vi "Harris Corner Detection.vi"() -> ()   [LabVIEW 2018]
doc: "Harris Corner Detection: This example is a Harris corner detection example, which can determine which pixels are corners based on the value of the corner response function by setting a threshold. If the corner response function value of a pixel is greater than the threshold and is a local maximum in its surrounding neighborhood, it is considered a corner."
uses:
  vi.lib/VIRobotics/opencv_yiku/ctls/ColorConversionCodes.ctl
  vi.lib/VIRobotics/opencv_yiku/Mat/Create_Mat_8U.vi
  vi.lib/VIRobotics/opencv_yiku/Mat/Mat_8U/set2ddata.vi
  vi.lib/VIRobotics/opencv_yiku/Mat/Mat_8U/Mat_8U.lvclass
  vi.lib/VIRobotics/opencv_yiku/opencv_yiku.lvlib
panel:
  out "max value":sgl
  out "corner":picture
  out "dst":sgl[][](array[numeric])
  out "picture":picture
  # "Overview: Demonstrates how to finish Harris Corner Detection\nRequirements: Windows.\nInstructions: \n1.Run the VI"
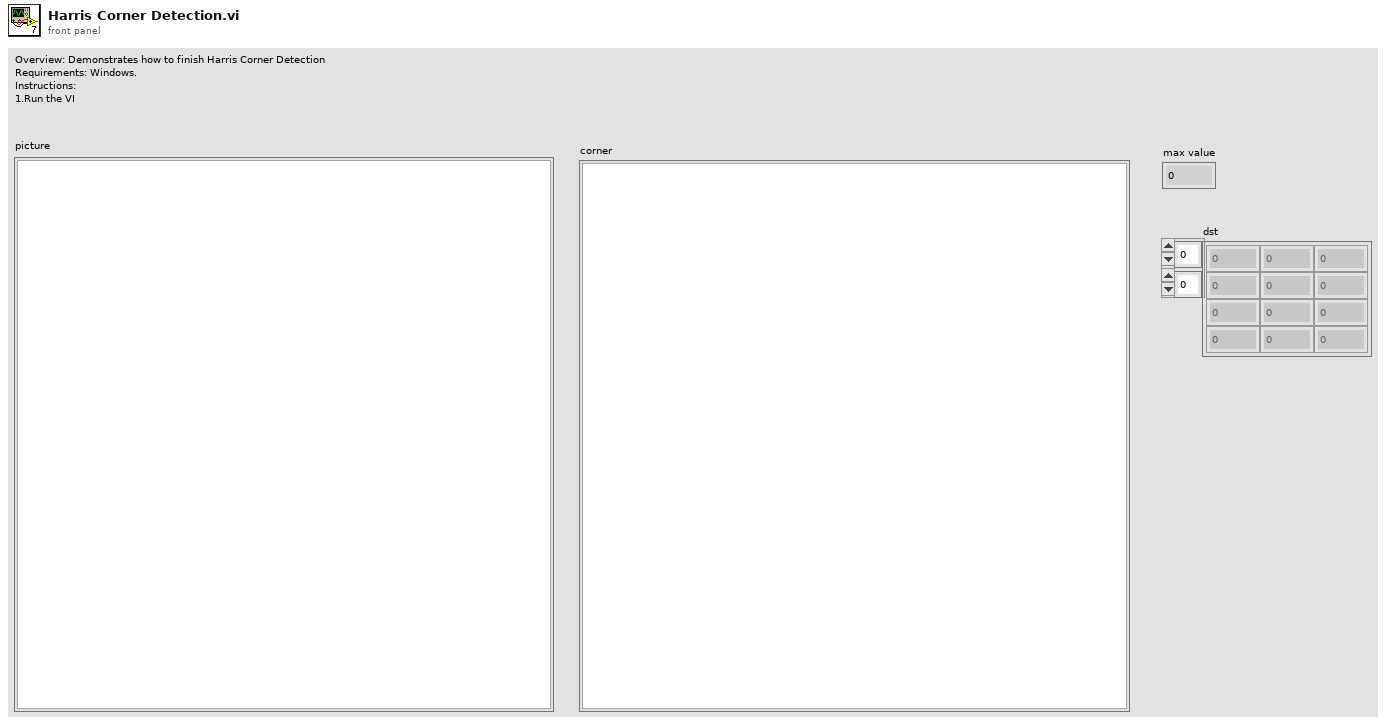
[diagram p1: front panel]
types:
  T1 = typedef "opencv_yiku.lvlib/ColorConversionCodes.ctl" = enum32{"COLOR_BGR2BGRA", "COLOR_BGRA2BGR", "COLOR_BGR2RGBA", "COLOR_RGBA2BGR", "COLOR_BGR2RGB", "COLOR_BGRA2RGBA", "COLOR_BGR2GRAY", "COLOR_RGB2GRAY", "COLOR_GRAY2BGR", "COLOR_GRAY2BGRA", "COLOR_BGRA2GRAY", "COLOR_RGBA2GRAY", "COLOR_BGR2BGR565", "COLOR_RGB2BGR565", "COLOR_BGR5652BGR", "COLOR_BGR5652RGB", "COLOR_BGRA2BGR565", "COLOR_RGBA2BGR565", "COLOR_BGR5652BGRA", "COLOR_BGR5652RGBA", "COLOR_GRAY2BGR565", "COLOR_BGR5652GRAY", "COLOR_BGR2BGR555", "COLOR_RGB2BGR555", "COLOR_BGR5552BGR", "COLOR_BGR5552RGB", "COLOR_BGRA2BGR555", "COLOR_RGBA2BGR555", "COLOR_BGR5552BGRA", "COLOR_BGR5552RGBA", "COLOR_GRAY2BGR555", "COLOR_BGR5552GRAY", "COLOR_BGR2XYZ", "COLOR_RGB2XYZ", "COLOR_XYZ2BGR", "COLOR_XYZ2RGB", "COLOR_BGR2YCrCb", "COLOR_RGB2YCrCb", "COLOR_YCrCb2BGR", "COLOR_YCrCb2RGB", "COLOR_BGR2HSV", "COLOR_RGB2HSV", "42", "43", "COLOR_BGR2Lab", "COLOR_RGB2Lab"}
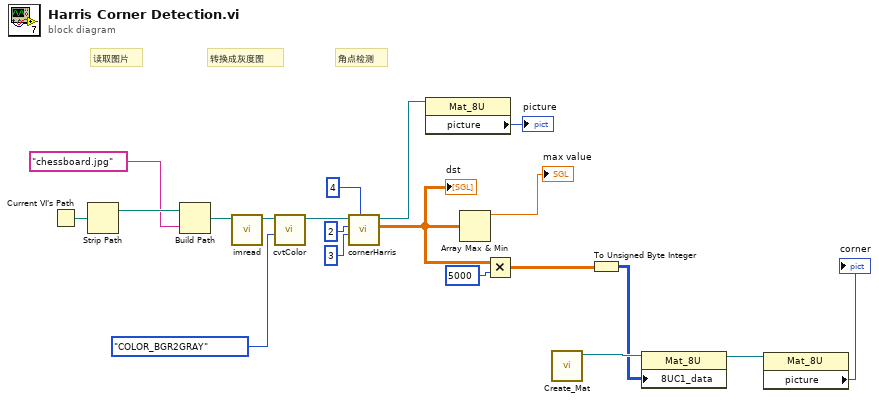
[diagram p0: block diagram]
diagram:
  # "角点检测"
  # "转换成灰度图"
  # "读取图片"
  n1 = Current VI's Path() -> (path=w19:path)
  n2 = Strip Path(path=w19) -> (stripped path=w20:path)  [unwired: 1 out]
  n3 = Build Path(base path=w20, name or relative path="chessboard.jpg") -> (appended path=w18:path)
  n4 = call "imread.vi"("path"=w18) -> ("Mat out"=w17:refnum<class "Mat_8U.lvclass">)  [unwired: 9 in, 1 out]
  n5 = call "cvtColor.vi"("dstCn"=ColorConversionCodes."COLOR_BGR2GRAY", "src"=w17) -> ("src out"=w15:refnum<class "Mat_8U.lvclass">)  [unwired: 7 in, 2 out]
  n6 = call "cornerHarris.vi"("borderType"=4, "ksize"=3, "blocksize"=2, "src"=w15) -> ("dst"=w8:sgl[][], "Mat out"=w14:refnum<class "Mat_8U.lvclass">)  [unwired: 5 in, 1 out]
  "dst" <- w8
  n7 = property class="Mat_8U"(reference=w14) -> ("picture"=→"picture":picture)  [unwired: 1 in, 2 out]
  n8 = Array Max & Min(array=w8) -> (max value=→"max value":sgl)  [unwired: 3 out]
  n9 = Multiply(x=w8, y=5000) -> (x*y=w9:sgl[][])
  n10 = call-poly "Create_Mat.vi"() -> ("Mat_8U_out"=w4:refnum<class "Mat_8U.lvclass">)  [unwired: 10 in, 1 out]
  n11 = To Unsigned Byte Integer(number=w9) -> (unsigned 8bit integer=w2:u8[][])
  n12 = property class="Mat_8U"(reference=w4, "8UC1_data"=w2) -> (reference out=w3:refnum<class "Mat_8U.lvclass">)  [unwired: 1 in, 1 out]
  n13 = property class="Mat_8U"(reference=w3) -> ("picture"=→"corner":picture)  [unwired: 1 in, 2 out]
